vi "At Least Identical Inputs.vi"(7 "Minimum Number of Calls":u32, 8 "error in (no error)":errorcluster, 11 "Mock in":refnum<class "LMock Mock.lvclass">) -> (0 "error out":errorcluster, 3 "Mock out":refnum<class "LMock Mock.lvclass">)   [LabVIEW 2020, in "Deprecated At Least.lvlib"]
doc: "This VI has been deprecated and will be removed in a future version of LMock. \nPlease use LMock At Least.vi instead."
uses:
  Deprecated At Least.lvlib
  Framework/Mock/LMock Mock.lvclass
  Comparators/Identical Inputs Comparator/Identical Inputs Comparator.lvclass
  C:/git/astemes-lmock/source/Core/Comparator/Comparator.lvclass
  At Least.lvclass
  C:/git/astemes-lmock/source/Core/Expectation/Expectation.lvclass
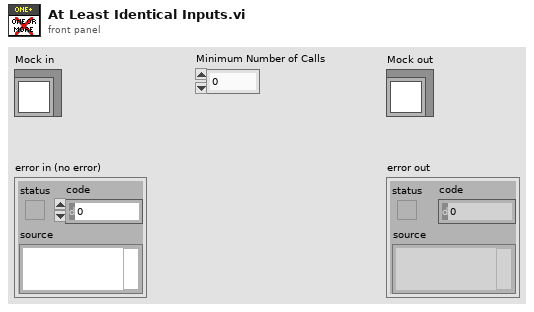
[diagram p1: front panel]
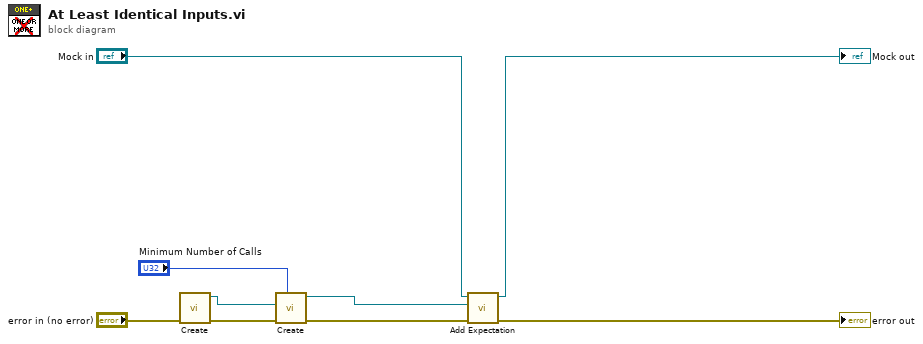
[diagram p0: block diagram]
diagram:
  n1 = call "Create.vi"("error in (no error)"="error in (no error)") -> ("error out"=w3:errorcluster, "Identical Inputs Comparator"=w2:refnum<class "Identical Inputs Comparator.lvclass">)  [unwired: 9 in]
  n2 = call "Create.vi"("Minimum Number of Calls"="Minimum Number of Calls", "error in (no error)"=w3, "Comparator"=w2) -> ("error out"=w5:errorcluster, "At Least Out"=w4:refnum<class "At Least.lvclass">)  [unwired: 7 in]
  n3 = call-dynamic "Add Expectation.vi"("error in (no error)"=w5, "Expectations"=w4, "Mock in"="Mock in") -> ("error out"=→"error out":errorcluster, "Mock out"=→"Mock out":refnum<class "LMock Mock.lvclass">)  [unwired: 7 in]
